vi "对中台复检判定.vi"(7 "Result":refnum<vi>, 10 "判定参数":T1={"主副信号和MAX"={"单位"="", "下限"=0.0, "上限"=0.0}, "主副信号和MIN"={"单位"="", "下限"=0.0, "上限"=0.0}, "主信号线性误差"={"单位"="", "下限"=0.0, "上限"=0.0}, "副信号线性误差"={"单位"="", "下限"=0.0, "上限"=0.0}, "主信号MAX"={"单位"="", "下限"=0.0, "上限"=0.0}, "主信号MIN"={"单位"="", "下限"=0.0, "上限"=0.0}, "副信号MAX"={"单位"="", "下限"=0.0, "上限"=0.0}, "副信号MIN"={"单位"="", "下限"=0.0, "上限"=0.0}, "中心偏移量"={"单位"="", "下限"=0.0, "上限"=0.0}, "定点设置"={"单位"="", "下限"=20.0, "上限"=30.0}, "定点左侧主信号"={"单位"="", "下限"=0.0, "上限"=0.0}, "定点左侧副信号"={"单位"="", "下限"=0.0, "上限"=0.0}, "定点右侧主信号"={"单位"="", "下限"=0.0, "上限"=0.0}, "定点右侧副信号"={"单位"="", "下限"=0.0, "上限"=0.0}, "监测点1主信号滞后"={"单位"="", "下限"=0.0, "上限"=0.0}, "监测点1副信号滞后"={"单位"="", "下限"=0.0, "上限"=0.0}, "监测点2主信号滞后"={"单位"="", "下限"=0.0, "上限"=0.0}, "监测点2副信号滞后"={"单位"="", "下限"=0.0, "上限"=0.0}, "监测点3主信号滞后"={"单位"="", "下限"=0.0, "上限"=0.0}, "监测点3副信号滞后"={"单位"="", "下限"=0.0, "上限"=0.0}}, 11 "XY曲线":cluster{"X":dbl[], "Y":dbl[]}[](array[cluster])) -> (3 "OK？":bool)   [LabVIEW 2020]
uses:
  <vilib>/Analysis/6fits.llb/Curve Fitting Criteria.ctl
  Global_Variable/Global.vi
  <vilib>/Analysis/NI_AALPro.lvlib
  <vilib>/Analysis/NI_AAL_Geometry.lvlib
panel:
  out "定点设置":dbl
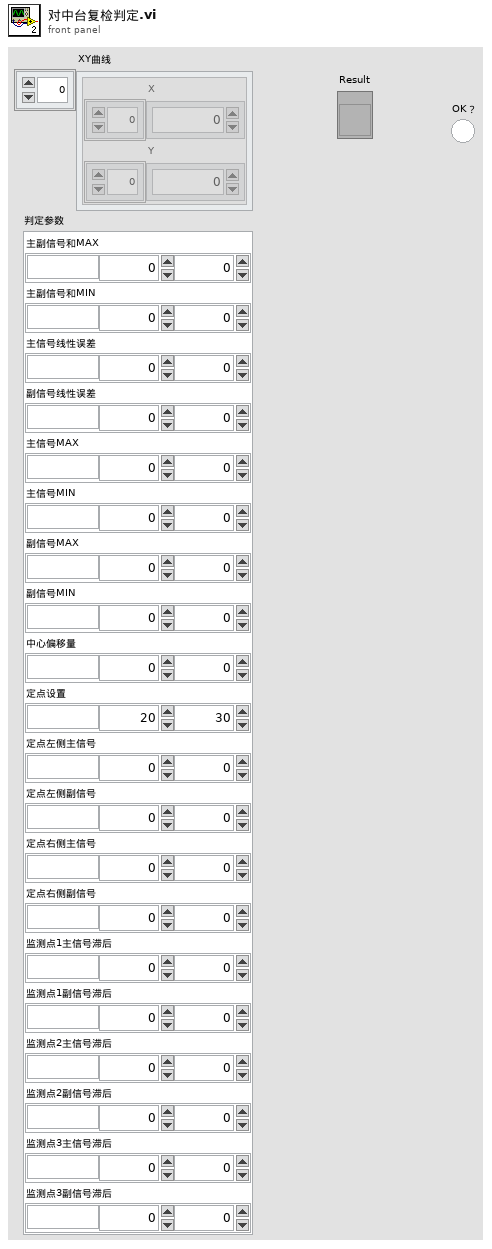
[diagram p1: front panel]
types:
  T1 = cluster{"主副信号和MAX":cluster{"单位":string, "下限":dbl, "上限":dbl}, "主副信号和MIN":cluster{"单位":string, "下限":dbl, "上限":dbl}, "主信号线性误差":cluster{"单位":string, "下限":dbl, "上限":dbl}, "副信号线性误差":cluster{"单位":string, "下限":dbl, "上限":dbl}, "主信号MAX":cluster{"单位":string, "下限":dbl, "上限":dbl}, "主信号MIN":cluster{"单位":string, "下限":dbl, "上限":dbl}, "副信号MAX":cluster{"单位":string, "下限":dbl, "上限":dbl}, "副信号MIN":cluster{"单位":string, "下限":dbl, "上限":dbl}, "中心偏移量":cluster{"单位":string, "下限":dbl, "上限":dbl}, "定点设置":cluster{"单位":string, "下限":dbl, "上限":dbl}, "定点左侧主信号":cluster{"单位":string, "下限":dbl, "上限":dbl}, "定点左侧副信号":cluster{"单位":string, "下限":dbl, "上限":dbl}, "定点右侧主信号":cluster{"单位":string, "下限":dbl, "上限":dbl}, "定点右侧副信号":cluster{"单位":string, "下限":dbl, "上限":dbl}, "监测点1主信号滞后":cluster{"单位":string, "下限":dbl, "上限":dbl}, "监测点1副信号滞后":cluster{"单位":string, "下限":dbl, "上限":dbl}, "监测点2主信号滞后":cluster{"单位":string, "下限":dbl, "上限":dbl}, "监测点2副信号滞后":cluster{"单位":string, "下限":dbl, "上限":dbl}, "监测点3主信号滞后":cluster{"单位":string, "下限":dbl, "上限":dbl}, "监测点3副信号滞后":cluster{"单位":string, "下限":dbl, "上限":dbl}}
  T2 = typedef "NI_AALPro.lvlib/Curve Fitting Criteria.ctl" = u16
  T3 = cluster{"复检速度":dbl, "换向扭矩":dbl, "判定范围下限":dbl, "判定范围上限":dbl, "滞后监测点1":dbl, "滞后监测点2":dbl, "滞后监测点3":dbl}
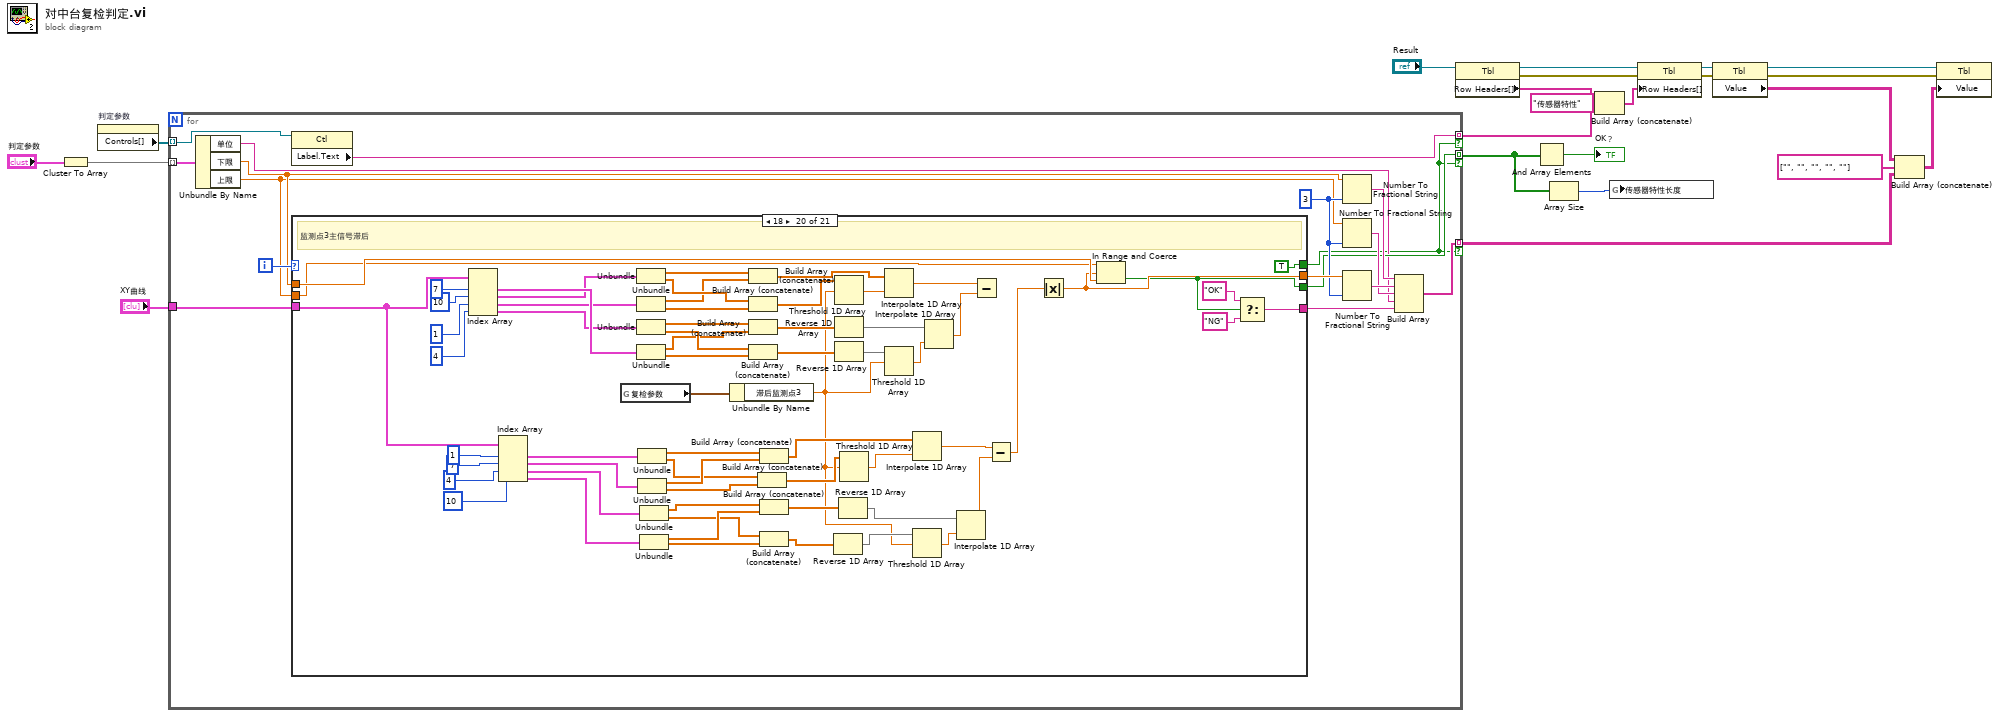
[diagram p0: block diagram]
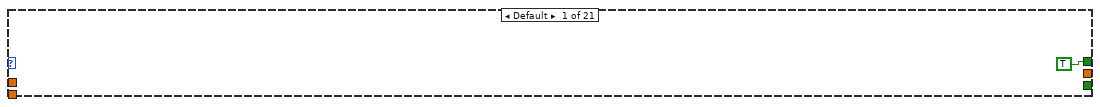
[diagram p2: hidden frame]
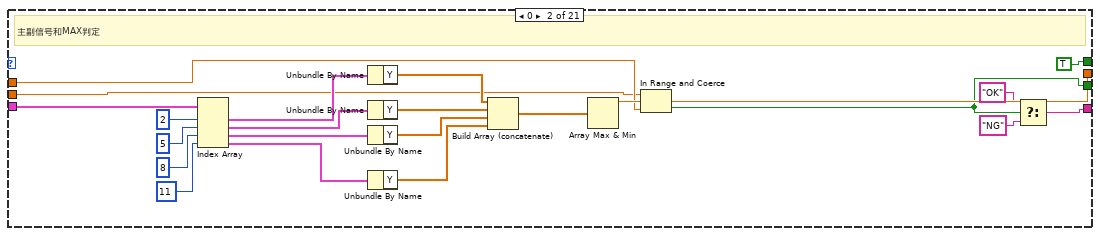
[diagram p3: hidden frame]
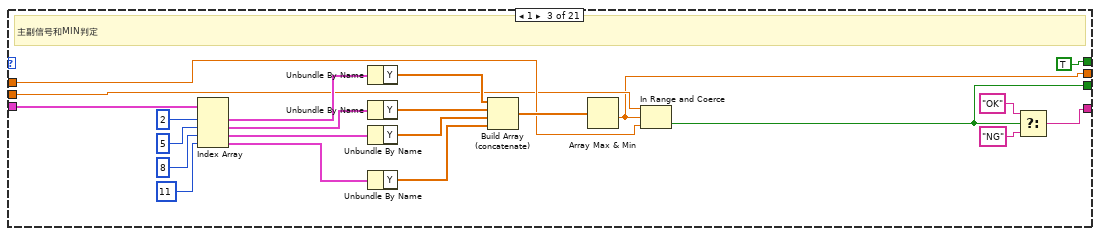
[diagram p4: hidden frame]
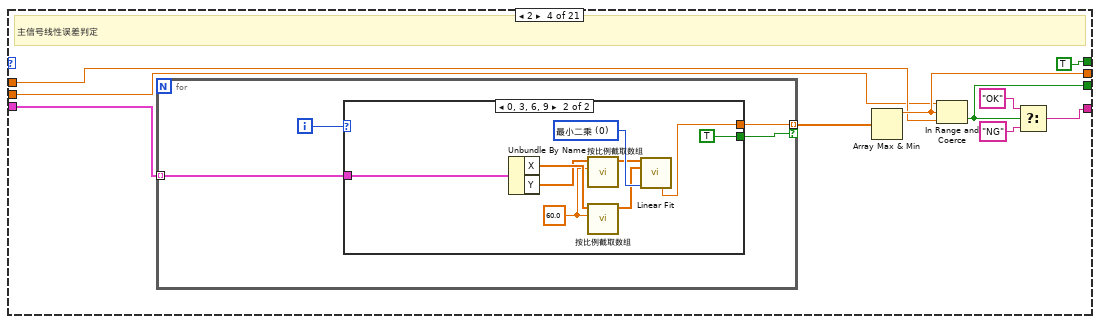
[diagram p5: hidden frame]
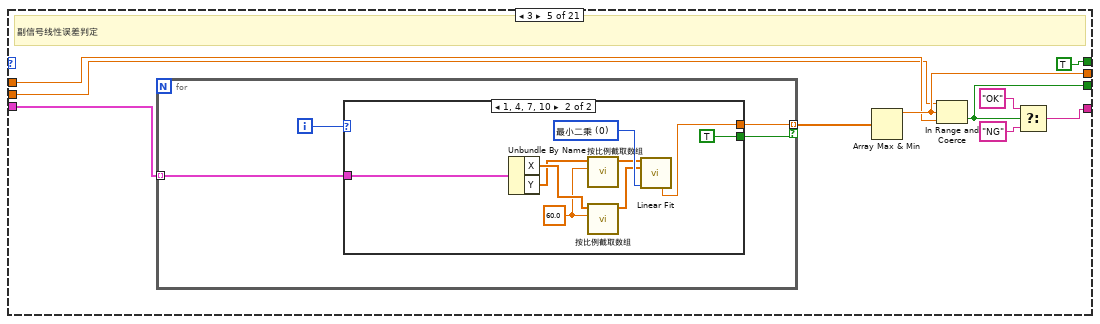
[diagram p7: hidden frame]
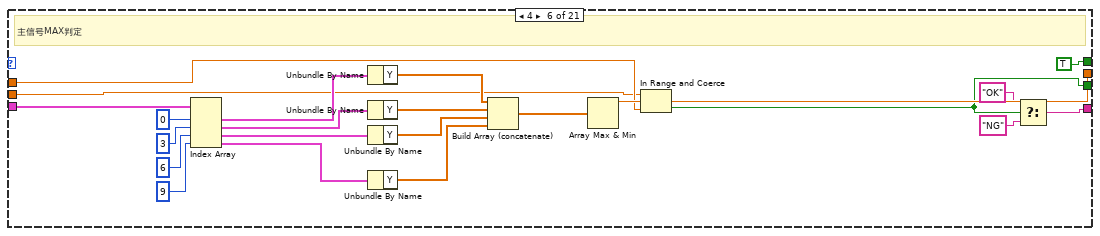
[diagram p9: hidden frame]
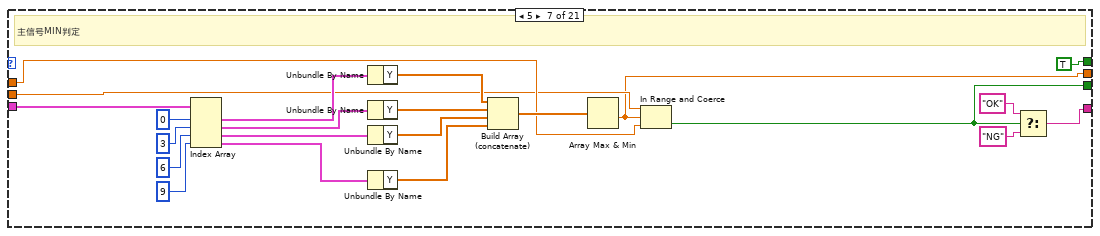
[diagram p10: hidden frame]
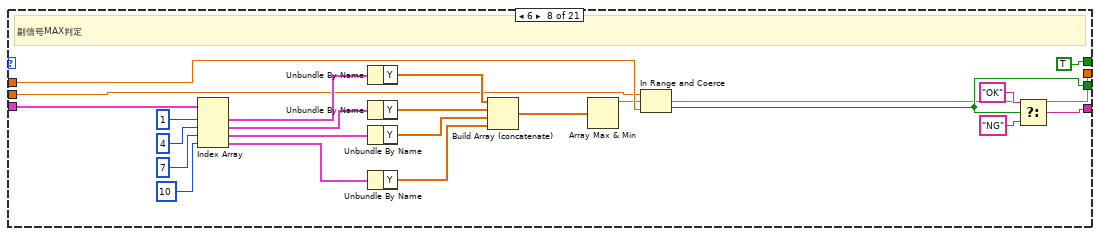
[diagram p11: hidden frame]
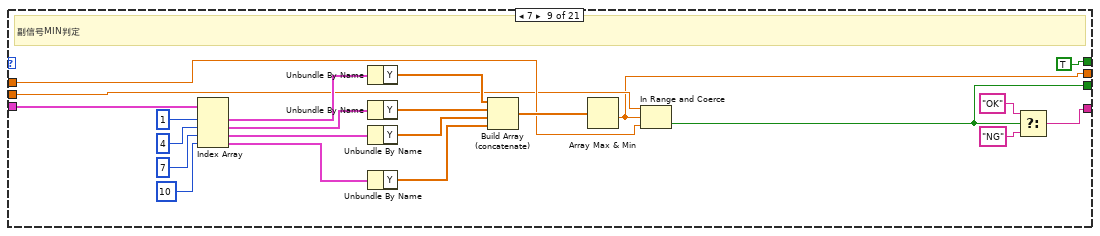
[diagram p12: hidden frame]
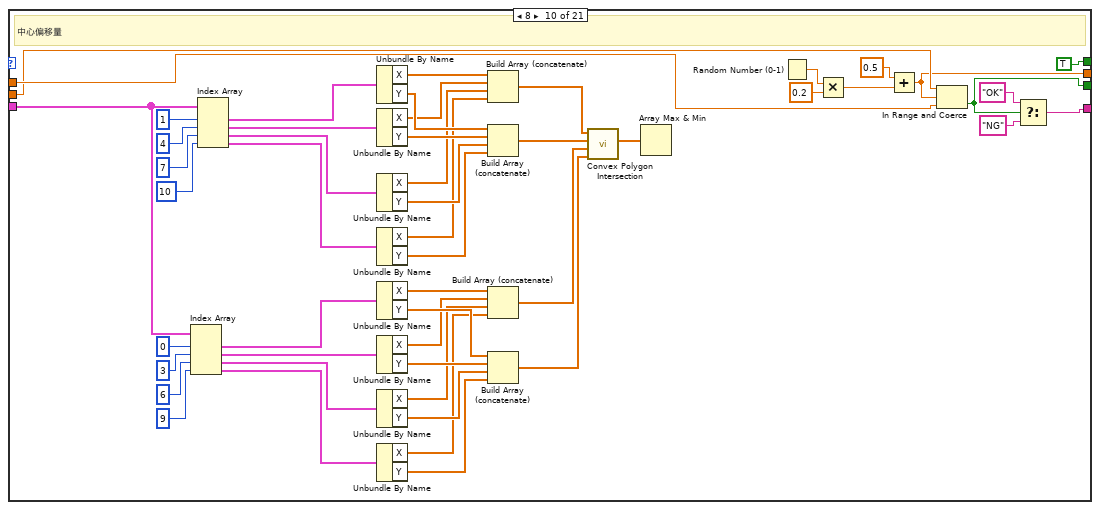
[diagram p13: hidden frame]
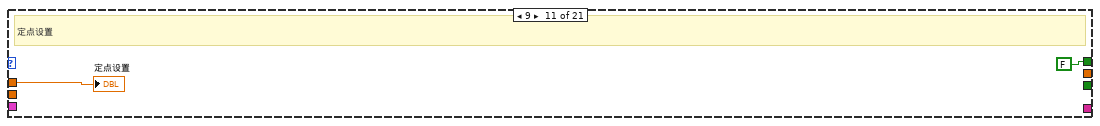
[diagram p14: hidden frame]
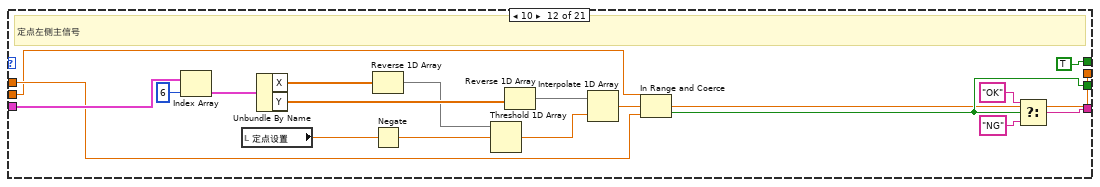
[diagram p15: hidden frame]
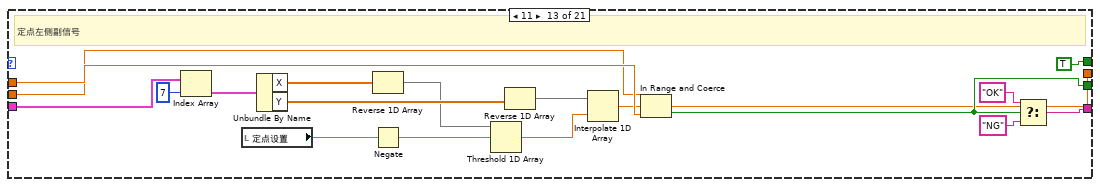
[diagram p16: hidden frame]
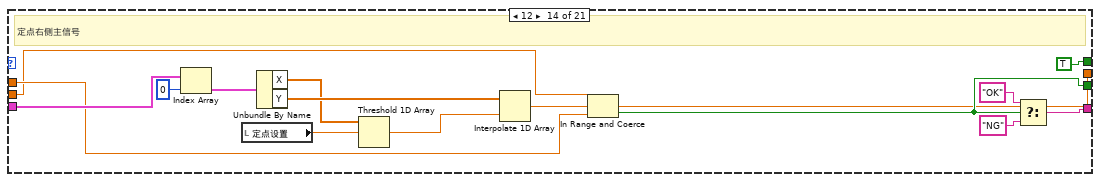
[diagram p17: hidden frame]
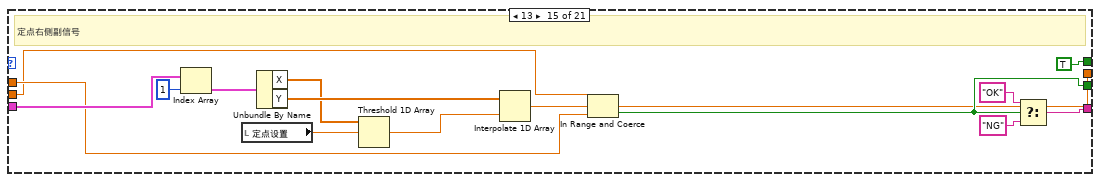
[diagram p18: hidden frame]
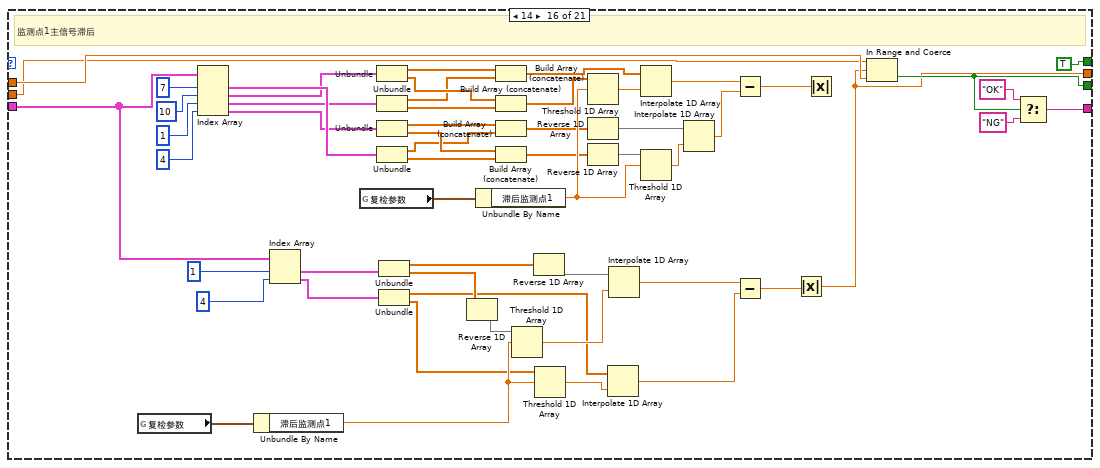
[diagram p19: hidden frame]
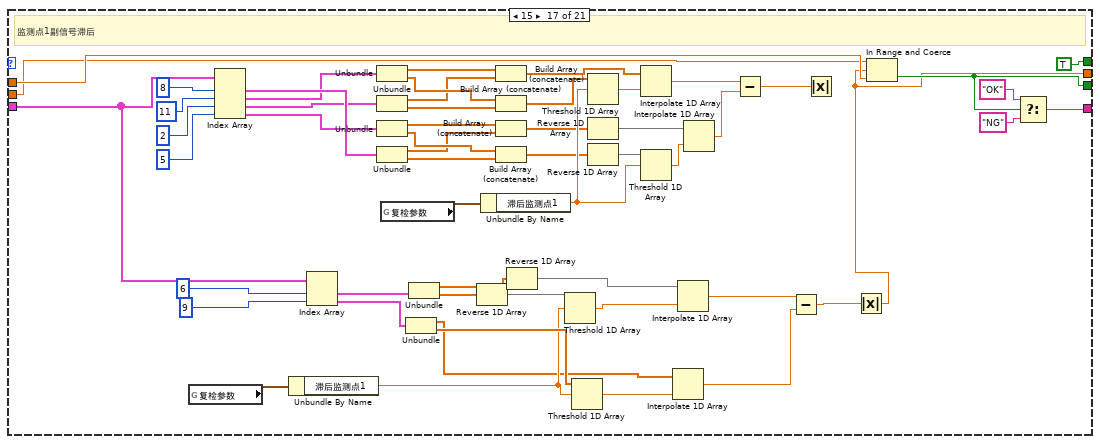
[diagram p20: hidden frame]
diagram:
  n1 = Cluster To Array(cluster="判定参数") -> (array=w22:cluster{"单位":string, "下限":dbl, "上限":dbl}[])
  n2 = property on="判定参数" class="Clust (严格)"() -> ("Controls[]"=w20:refnum<vi>[])  [unwired: 2 in, 2 out]
  n3 = for {
    tunnel: w22 -> [w39] mode=indexing
    tunnel: w20 -> [w37] mode=indexing
    tunnel: "XY曲线" -> [w35]
    tunnel: [w29] -> w2 mode=indexing if=w23
    tunnel: [w25] -> w4 mode=indexing if=w23
    tunnel: [w24] -> w8 mode=indexing if=w23
    i -> [w38]
    w34 = i16 3 ("精度(6)")
    n4 = Unbundle By Name(w39) -> ("单位"=w28:string, "下限"=w27:dbl, "上限"=w26:dbl)
    n5 = property class="Ctl"(reference=w37) -> ("Label.Text"=w24:string)  [unwired: 1 in, 2 out]
    n6 = case shown="18" w38 {
      tunnel: [_ w48 w63 w94 w117 w138 w154 w176 w198 w219 _ w275 w292 w309 w324 w340 w392 w447 w500 w607 w643] -> w36
      tunnel: w35 -> [_ w62 w84 w86 w109 w152 w174 w196 w218 w237 _ w288 w306 w321 w336 w355 w410 w457 w504 w581 w621]
      tunnel: [_ w45 w68 w91 w114 w135 w158 w180 w202 w254 _ w284 w302 w317 w332 w377 w432 w486 w539 w603 w639] -> w30
      tunnel: [_ w44 w67 w90 w113 w134 w157 w179 w201 w253 _ w283 w301 w316 w331 w378 w433 w487 w540 w604 w640] -> w29
      tunnel: w27 -> [_ w43 w66 w89 w112 w133 w156 w178 w200 w252 w269 w282 w300 w315 w330 w382 w437 w491 w544 w609 w645]
      tunnel: w26 -> [_ w42 w65 w88 w111 w132 w155 w177 w199 w251 _ w281 w299 w314 w329 w381 w436 w490 w543 w608 w644]
      tunnel: [TRUE TRUE TRUE TRUE TRUE TRUE TRUE TRUE TRUE TRUE FALSE TRUE TRUE TRUE TRUE TRUE TRUE TRUE TRUE TRUE TRUE] -> w23
      frame Default {
      }
      frame 0 {
        # "主副信号和MAX判定"
        n7 = Index Array(array=w62, index #1=2 ("索引"), index #2=5 ("索引"), index #3=8 ("索引"), index #4=11 ("索引")) -> (element #1=w57:cluster{"X":dbl[], "Y":dbl[]}, element #2=w54:cluster{"X":dbl[], "Y":dbl[]}, element #3=w55:cluster{"X":dbl[], "Y":dbl[]}, element #4=w56:cluster{"X":dbl[], "Y":dbl[]})
        n8 = Unbundle By Name(w57) -> ("Y"=w53:dbl[])
        n9 = Unbundle By Name(w54) -> ("Y"=w52:dbl[])
        n10 = Unbundle By Name(w55) -> ("Y"=w51:dbl[])
        n11 = Unbundle By Name(w56) -> ("Y"=w50:dbl[])
        n12 = Build Array (concatenate)(w53, w52, w51, w50) -> (w49:dbl[])
        n13 = Array Max & Min(array=w49) -> (max value=w48:dbl)  [unwired: 3 out]
        n14 = In Range and Coerce(upper limit=w42, x=w48, lower limit=w43) -> (In Range?=w44:bool)  [unwired: 1 out]
        n15 = Select(t="OK", s=w44, f="NG") -> (s? t:f=w45:string)
      }
      frame 1 {
        # "主副信号和MIN判定"
        n16 = Index Array(array=w84, index #1=2 ("索引"), index #2=5 ("索引"), index #3=8 ("索引"), index #4=11 ("索引")) -> (element #1=w79:cluster{"X":dbl[], "Y":dbl[]}, element #2=w76:cluster{"X":dbl[], "Y":dbl[]}, element #3=w77:cluster{"X":dbl[], "Y":dbl[]}, element #4=w78:cluster{"X":dbl[], "Y":dbl[]})
        n17 = Unbundle By Name(w79) -> ("Y"=w75:dbl[])
        n18 = Unbundle By Name(w76) -> ("Y"=w74:dbl[])
        n19 = Unbundle By Name(w77) -> ("Y"=w73:dbl[])
        n20 = Unbundle By Name(w78) -> ("Y"=w72:dbl[])
        n21 = Build Array (concatenate)(w75, w74, w73, w72) -> (w71:dbl[])
        n22 = Array Max & Min(array=w71) -> (min value=w63:dbl)  [unwired: 3 out]
        n23 = In Range and Coerce(upper limit=w65, x=w63, lower limit=w66) -> (In Range?=w67:bool)  [unwired: 1 out]
        n24 = Select(t="OK", s=w67, f="NG") -> (s? t:f=w68:string)
      }
      frame 2 {
        # "主信号线性误差判定"
        n25 = for {
          tunnel: w86 -> [w97] mode=indexing
          tunnel: [w96] -> w85 mode=indexing if=w95
          i -> [w98]
          n26 = case shown="0, 3, 6, 9" w98 {
            tunnel: w97 -> [_ w107]
            tunnel: [_ w105] -> w96
            tunnel: [_ TRUE] -> w95
            frame Default {
            }
            frame 0, 3, 6, 9 {
              w99 = 60.0 ("长度")
              w106 = T2 0 items=["最小二乘", "最小绝对残差", "Bisquare"] ("method")
              n27 = Unbundle By Name(w107) -> ("X"=w103:dbl[], "Y"=w101:dbl[])
              n28 = call "按比例截取数组.vi"("长度"=w99, "X"=w101) -> ("Y"=w100:dbl[])  [unwired: 9 in]
              n29 = call "按比例截取数组.vi"("长度"=w99, "X"=w103) -> ("Y"=w102:dbl[])  [unwired: 9 in]
              n30 = call <vilib>:"Linear Fit.vi"("Y"=w100, "X"=w102, "method"=w106) -> ("residue"=w105:dbl)  [unwired: 8 in, 4 out]
            }
          }
        }
        n31 = Array Max & Min(array=w85) -> (max value=w94:dbl)  [unwired: 3 out]
        n32 = In Range and Coerce(upper limit=w88, x=w94, lower limit=w89) -> (In Range?=w90:bool)  [unwired: 1 out]
        n33 = Select(t="OK", s=w90, f="NG") -> (s? t:f=w91:string)
      }
      frame 3 {
        # "副信号线性误差判定"
        n34 = for {
          tunnel: w109 -> [w120] mode=indexing
          tunnel: [w119] -> w108 mode=indexing if=w118
          i -> [w121]
          n35 = case shown="1, 4, 7, 10" w121 {
            tunnel: w120 -> [_ w130]
            tunnel: [_ w128] -> w119
            tunnel: [_ TRUE] -> w118
            frame Default {
            }
            frame 1, 4, 7, 10 {
              w122 = 60.0 ("长度")
              w129 = T2 0 items=["最小二乘", "最小绝对残差", "Bisquare"] ("method")
              n36 = Unbundle By Name(w130) -> ("X"=w126:dbl[], "Y"=w124:dbl[])
              n37 = call "按比例截取数组.vi"("长度"=w122, "X"=w124) -> ("Y"=w123:dbl[])  [unwired: 9 in]
              n38 = call "按比例截取数组.vi"("长度"=w122, "X"=w126) -> ("Y"=w125:dbl[])  [unwired: 9 in]
              n39 = call <vilib>:"Linear Fit.vi"("Y"=w123, "X"=w125, "method"=w129) -> ("residue"=w128:dbl)  [unwired: 8 in, 4 out]
            }
          }
        }
        n40 = Array Max & Min(array=w108) -> (max value=w117:dbl)  [unwired: 3 out]
        n41 = In Range and Coerce(upper limit=w111, x=w117, lower limit=w112) -> (In Range?=w113:bool)  [unwired: 1 out]
        n42 = Select(t="OK", s=w113, f="NG") -> (s? t:f=w114:string)
      }
      frame 4 {
        # "主信号MAX判定"
        n43 = Index Array(array=w152, index #1=0 ("索引"), index #2=3 ("索引"), index #3=6 ("索引"), index #4=9 ("索引")) -> (element #1=w147:cluster{"X":dbl[], "Y":dbl[]}, element #2=w144:cluster{"X":dbl[], "Y":dbl[]}, element #3=w145:cluster{"X":dbl[], "Y":dbl[]}, element #4=w146:cluster{"X":dbl[], "Y":dbl[]})
        n44 = Unbundle By Name(w147) -> ("Y"=w143:dbl[])
        n45 = Unbundle By Name(w144) -> ("Y"=w142:dbl[])
        n46 = Unbundle By Name(w145) -> ("Y"=w141:dbl[])
        n47 = Unbundle By Name(w146) -> ("Y"=w140:dbl[])
        n48 = Build Array (concatenate)(w143, w142, w141, w140) -> (w139:dbl[])
        n49 = Array Max & Min(array=w139) -> (max value=w138:dbl)  [unwired: 3 out]
        n50 = In Range and Coerce(upper limit=w132, x=w138, lower limit=w133) -> (In Range?=w134:bool)  [unwired: 1 out]
        n51 = Select(t="OK", s=w134, f="NG") -> (s? t:f=w135:string)
      }
      frame 5 {
        # "主信号MIN判定"
        n52 = Index Array(array=w174, index #1=0 ("索引"), index #2=3 ("索引"), index #3=6 ("索引"), index #4=9 ("索引")) -> (element #1=w169:cluster{"X":dbl[], "Y":dbl[]}, element #2=w166:cluster{"X":dbl[], "Y":dbl[]}, element #3=w167:cluster{"X":dbl[], "Y":dbl[]}, element #4=w168:cluster{"X":dbl[], "Y":dbl[]})
        n53 = Unbundle By Name(w169) -> ("Y"=w165:dbl[])
        n54 = Unbundle By Name(w166) -> ("Y"=w164:dbl[])
        n55 = Unbundle By Name(w167) -> ("Y"=w163:dbl[])
        n56 = Unbundle By Name(w168) -> ("Y"=w162:dbl[])
        n57 = Build Array (concatenate)(w165, w164, w163, w162) -> (w161:dbl[])
        n58 = Array Max & Min(array=w161) -> (min value=w154:dbl)  [unwired: 3 out]
        n59 = In Range and Coerce(upper limit=w155, x=w154, lower limit=w156) -> (In Range?=w157:bool)  [unwired: 1 out]
        n60 = Select(t="OK", s=w157, f="NG") -> (s? t:f=w158:string)
      }
      frame 6 {
        # "副信号MAX判定"
        n61 = Index Array(array=w196, index #1=1 ("索引"), index #2=4 ("索引"), index #3=7 ("索引"), index #4=10 ("索引")) -> (element #1=w191:cluster{"X":dbl[], "Y":dbl[]}, element #2=w188:cluster{"X":dbl[], "Y":dbl[]}, element #3=w189:cluster{"X":dbl[], "Y":dbl[]}, element #4=w190:cluster{"X":dbl[], "Y":dbl[]})
        n62 = Unbundle By Name(w191) -> ("Y"=w187:dbl[])
        n63 = Unbundle By Name(w188) -> ("Y"=w186:dbl[])
        n64 = Unbundle By Name(w189) -> ("Y"=w185:dbl[])
        n65 = Unbundle By Name(w190) -> ("Y"=w184:dbl[])
        n66 = Build Array (concatenate)(w187, w186, w185, w184) -> (w183:dbl[])
        n67 = Array Max & Min(array=w183) -> (max value=w176:dbl)  [unwired: 3 out]
        n68 = In Range and Coerce(upper limit=w177, x=w176, lower limit=w178) -> (In Range?=w179:bool)  [unwired: 1 out]
        n69 = Select(t="OK", s=w179, f="NG") -> (s? t:f=w180:string)
      }
      frame 7 {
        # "副信号MIN判定"
        n70 = Index Array(array=w218, index #1=1 ("索引"), index #2=4 ("索引"), index #3=7 ("索引"), index #4=10 ("索引")) -> (element #1=w213:cluster{"X":dbl[], "Y":dbl[]}, element #2=w210:cluster{"X":dbl[], "Y":dbl[]}, element #3=w211:cluster{"X":dbl[], "Y":dbl[]}, element #4=w212:cluster{"X":dbl[], "Y":dbl[]})
        n71 = Unbundle By Name(w213) -> ("Y"=w209:dbl[])
        n72 = Unbundle By Name(w210) -> ("Y"=w208:dbl[])
        n73 = Unbundle By Name(w211) -> ("Y"=w207:dbl[])
        n74 = Unbundle By Name(w212) -> ("Y"=w206:dbl[])
        n75 = Build Array (concatenate)(w209, w208, w207, w206) -> (w205:dbl[])
        n76 = Array Max & Min(array=w205) -> (min value=w198:dbl)  [unwired: 3 out]
        n77 = In Range and Coerce(upper limit=w199, x=w198, lower limit=w200) -> (In Range?=w201:bool)  [unwired: 1 out]
        n78 = Select(t="OK", s=w201, f="NG") -> (s? t:f=w202:string)
      }
      frame 8 {
        # "中心偏移量"
        n79 = Index Array(array=w237, index #1=0 ("索引"), index #2=3 ("索引"), index #3=6 ("索引"), index #4=9 ("索引")) -> (element #1=w264:cluster{"X":dbl[], "Y":dbl[]}, element #2=w261:cluster{"X":dbl[], "Y":dbl[]}, element #3=w262:cluster{"X":dbl[], "Y":dbl[]}, element #4=w263:cluster{"X":dbl[], "Y":dbl[]})
        n80 = Index Array(array=w237, index #1=1 ("索引"), index #2=4 ("索引"), index #3=7 ("索引"), index #4=10 ("索引")) -> (element #1=w242:cluster{"X":dbl[], "Y":dbl[]}, element #2=w245:cluster{"X":dbl[], "Y":dbl[]}, element #3=w244:cluster{"X":dbl[], "Y":dbl[]}, element #4=w243:cluster{"X":dbl[], "Y":dbl[]})
        n81 = Unbundle By Name(w242) -> ("X"=w236:dbl[], "Y"=w246:dbl[])
        n82 = Unbundle By Name(w245) -> ("X"=w235:dbl[], "Y"=w247:dbl[])
        n83 = Unbundle By Name(w244) -> ("X"=w234:dbl[], "Y"=w248:dbl[])
        n84 = Unbundle By Name(w243) -> ("X"=w233:dbl[], "Y"=w249:dbl[])
        n85 = Unbundle By Name(w264) -> ("X"=w232:dbl[], "Y"=w260:dbl[])
        n86 = Unbundle By Name(w261) -> ("X"=w231:dbl[], "Y"=w259:dbl[])
        n87 = Unbundle By Name(w262) -> ("X"=w230:dbl[], "Y"=w258:dbl[])
        n88 = Unbundle By Name(w263) -> ("X"=w229:dbl[], "Y"=w257:dbl[])
        n89 = Build Array (concatenate)(w236, w235, w234, w233) -> (w226:dbl[])
        n90 = Build Array (concatenate)(w246, w247, w248, w249) -> (w228:dbl[])
        n91 = Build Array (concatenate)(w232, w231, w230, w229) -> (w225:dbl[])
        n92 = Build Array (concatenate)(w260, w259, w258, w257) -> (w224:dbl[])
        n93 = call <vilib>:"Convex Polygon Intersection.vi"("Y 2"=w224, "X 2"=w225, "Y 1"=w228, "X 1"=w226) -> ("Intersection Y"=w227:dbl[])  [unwired: 5 in, 2 out]
        n94 = Array Max & Min(array=w227) -> ()  [unwired: 4 out]
        n95 = Random Number (0-1)() -> (number: 0 to 1=w222:dbl)
        n96 = Multiply(x=w222, y=0.2) -> (x*y=w220:dbl)
        n97 = Add(x=0.5, y=w220) -> (x+y=w219:dbl)
        n98 = In Range and Coerce(upper limit=w251, x=w219, lower limit=w252) -> (In Range?=w253:bool)  [unwired: 1 out]
        n99 = Select(t="OK", s=w253, f="NG") -> (s? t:f=w254:string)
      }
      frame 9 {
        # "定点设置"
        "定点设置" <- w269
      }
      frame 10 {
        # "定点左侧主信号"
        n100 = Index Array(array=w288, index=6 ("索引")) -> (element=w287:cluster{"X":dbl[], "Y":dbl[]})
        n101 = local read "定点设置"() -> (w277:dbl)
        n102 = Unbundle By Name(w287) -> ("X"=w274:dbl[], "Y"=w276:dbl[])
        n103 = Reverse 1D Array(array=w274) -> (reversed array=w272:dbl[])
        n104 = Negate(x=w277) -> (-x=w273:dbl)
        n105 = Threshold 1D Array(2:w273, 3:w272) -> (0:w278:dbl)  [unwired: 1 in]
        n106 = Reverse 1D Array(array=w276) -> (reversed array=w271:dbl[])
        n107 = Interpolate 1D Array(1:w278, 2:w271) -> (0:w275:dbl)
        n108 = In Range and Coerce(upper limit=w281, x=w275, lower limit=w282) -> (In Range?=w283:bool)  [unwired: 1 out]
        n109 = Select(t="OK", s=w283, f="NG") -> (s? t:f=w284:string)
      }
      frame 11 {
        # "定点左侧副信号"
        n110 = Index Array(array=w306, index=7 ("索引")) -> (element=w305:cluster{"X":dbl[], "Y":dbl[]})
        n111 = local read "定点设置"() -> (w294:dbl)
        n112 = Unbundle By Name(w305) -> ("X"=w295:dbl[], "Y"=w293:dbl[])
        n113 = Reverse 1D Array(array=w295) -> (reversed array=w291:dbl[])
        n114 = Negate(x=w294) -> (-x=w289:dbl)
        n115 = Threshold 1D Array(2:w289, 3:w291) -> (0:w296:dbl)  [unwired: 1 in]
        n116 = Reverse 1D Array(array=w293) -> (reversed array=w290:dbl[])
        n117 = Interpolate 1D Array(1:w296, 2:w290) -> (0:w292:dbl)
        n118 = In Range and Coerce(upper limit=w299, x=w292, lower limit=w300) -> (In Range?=w301:bool)  [unwired: 1 out]
        n119 = Select(t="OK", s=w301, f="NG") -> (s? t:f=w302:string)
      }
      frame 12 {
        # "定点右侧主信号"
        n120 = Index Array(array=w321, index=0 ("索引")) -> (element=w320:cluster{"X":dbl[], "Y":dbl[]})
        n121 = local read "定点设置"() -> (w307:dbl)
        n122 = Unbundle By Name(w320) -> ("X"=w308:dbl[], "Y"=w310:dbl[])
        n123 = Threshold 1D Array(2:w307, 3:w308) -> (0:w311:dbl)  [unwired: 1 in]
        n124 = Interpolate 1D Array(1:w311, 2:w310) -> (0:w309:dbl)
        n125 = In Range and Coerce(upper limit=w314, x=w309, lower limit=w315) -> (In Range?=w316:bool)  [unwired: 1 out]
        n126 = Select(t="OK", s=w316, f="NG") -> (s? t:f=w317:string)
      }
      frame 13 {
        # "定点右侧副信号"
        n127 = Index Array(array=w336, index=1 ("索引")) -> (element=w335:cluster{"X":dbl[], "Y":dbl[]})
        n128 = local read "定点设置"() -> (w322:dbl)
        n129 = Unbundle By Name(w335) -> ("X"=w323:dbl[], "Y"=w325:dbl[])
        n130 = Threshold 1D Array(2:w322, 3:w323) -> (0:w326:dbl)  [unwired: 1 in]
        n131 = Interpolate 1D Array(1:w326, 2:w325) -> (0:w324:dbl)
        n132 = In Range and Coerce(upper limit=w329, x=w324, lower limit=w330) -> (In Range?=w331:bool)  [unwired: 1 out]
        n133 = Select(t="OK", s=w331, f="NG") -> (s? t:f=w332:string)
      }
      frame 14 {
        # "监测点1主信号滞后"
        n134 = global read "Global.vi" "复检参数"() -> (w350:T3)
        n135 = Index Array(array=w355, index #1=7 ("索引"), index #2=10 ("索引"), index #3=1 ("索引"), index #4=4 ("索引")) -> (element #1=w373:cluster{"X":dbl[], "Y":dbl[]}, element #2=w372:cluster{"X":dbl[], "Y":dbl[]}, element #3=w369:cluster{"X":dbl[], "Y":dbl[]}, element #4=w368:cluster{"X":dbl[], "Y":dbl[]})
        n136 = Unbundle By Name(w350) -> ("滞后监测点1"=w347:dbl)
        n137 = Index Array(array=w355, index #1=1 ("索引"), index #2=4 ("索引")) -> (element #1=w352:cluster{"X":dbl[], "Y":dbl[]}, element #2=w351:cluster{"X":dbl[], "Y":dbl[]})
        n138 = global read "Global.vi" "复检参数"() -> (w391:T3)
        n139 = Unbundle(w372) -> ("X"=w367:dbl[], "Y"=w366:dbl[])
        n140 = Unbundle(w369) -> ("X"=w365:dbl[], "Y"=w364:dbl[])
        n141 = Unbundle(w368) -> ("X"=w363:dbl[], "Y"=w362:dbl[])
        n142 = Unbundle(w373) -> ("X"=w361:dbl[], "Y"=w360:dbl[])
        n143 = Unbundle(w352) -> ("X"=w343:dbl[], "Y"=w342:dbl[])
        n144 = Unbundle(w351) -> ("X"=w339:dbl[], "Y"=w341:dbl[])
        n145 = Reverse 1D Array(array=w342) -> (reversed array=w337:dbl[])
        n146 = Unbundle By Name(w391) -> ("滞后监测点1"=w388:dbl)
        n147 = Build Array (concatenate)(w367, w365) -> (w359:dbl[])
        n148 = Build Array (concatenate)(w366, w364) -> (w358:dbl[])
        n149 = Build Array (concatenate)(w363, w361) -> (w357:dbl[])
        n150 = Build Array (concatenate)(w362, w360) -> (w356:dbl[])
        n151 = Threshold 1D Array(2:w347, 3:w337) -> (0:w349:dbl)  [unwired: 1 in]
        n152 = Reverse 1D Array(array=w343) -> (reversed array=w338:dbl[])
        n153 = Threshold 1D Array(2:w347, 3:w341) -> (0:w345:dbl)  [unwired: 1 in]
        n154 = Threshold 1D Array(2:w388, 3:w358) -> (0:w390:dbl)  [unwired: 1 in]
        n155 = Reverse 1D Array(array=w357) -> (reversed array=w376:dbl[])
        n156 = Reverse 1D Array(array=w356) -> (reversed array=w389:dbl[])
        n157 = Interpolate 1D Array(1:w345, 2:w339) -> (0:w344:dbl)
        n158 = Interpolate 1D Array(1:w349, 2:w338) -> (0:w348:dbl)
        n159 = Interpolate 1D Array(1:w390, 2:w359) -> (0:w386:dbl)
        n160 = Threshold 1D Array(2:w388, 3:w389) -> (0:w387:dbl)  [unwired: 1 in]
        n161 = Interpolate 1D Array(1:w387, 2:w376) -> (0:w385:dbl)
        n162 = Subtract(x=w386, y=w385) -> (x-y=w384:dbl)
        n163 = Subtract(x=w348, y=w344) -> (x-y=w346:dbl)
        n164 = Absolute Value(x=w346) -> (abs(x)=w340:dbl)
        n165 = Absolute Value(x=w384) -> ()  [unwired: 1 out]
        n166 = In Range and Coerce(upper limit=w381, x=w340, lower limit=w382) -> (In Range?=w378:bool)  [unwired: 1 out]
        n167 = Select(t="OK", s=w378, f="NG") -> (s? t:f=w377:string)
      }
      frame 15 {
        # "监测点1副信号滞后"
        n168 = global read "Global.vi" "复检参数"() -> (w405:T3)
        n169 = Index Array(array=w410, index #1=8 ("索引"), index #2=11 ("索引"), index #3=2 ("索引"), index #4=5 ("索引")) -> (element #1=w428:cluster{"X":dbl[], "Y":dbl[]}, element #2=w427:cluster{"X":dbl[], "Y":dbl[]}, element #3=w424:cluster{"X":dbl[], "Y":dbl[]}, element #4=w423:cluster{"X":dbl[], "Y":dbl[]})
        n170 = Unbundle By Name(w405) -> ("滞后监测点1"=w399:dbl)
        n171 = Index Array(array=w410, index #1=6 ("索引"), index #2=9 ("索引")) -> (element #1=w407:cluster{"X":dbl[], "Y":dbl[]}, element #2=w406:cluster{"X":dbl[], "Y":dbl[]})
        n172 = Unbundle(w427) -> ("X"=w422:dbl[], "Y"=w421:dbl[])
        n173 = Unbundle(w424) -> ("X"=w420:dbl[], "Y"=w419:dbl[])
        n174 = Unbundle(w423) -> ("X"=w418:dbl[], "Y"=w417:dbl[])
        n175 = Unbundle(w428) -> ("X"=w416:dbl[], "Y"=w415:dbl[])
        n176 = global read "Global.vi" "复检参数"() -> (w446:T3)
        n177 = Unbundle(w406) -> ("X"=w395:dbl[], "Y"=w400:dbl[])
        n178 = Unbundle(w407) -> ("X"=w403:dbl[], "Y"=w404:dbl[])
        n179 = Reverse 1D Array(array=w404) -> (reversed array=w393:dbl[])
        n180 = Unbundle By Name(w446) -> ("滞后监测点1"=w443:dbl)
        n181 = Build Array (concatenate)(w422, w420) -> (w414:dbl[])
        n182 = Build Array (concatenate)(w421, w419) -> (w413:dbl[])
        n183 = Build Array (concatenate)(w418, w416) -> (w412:dbl[])
        n184 = Build Array (concatenate)(w417, w415) -> (w411:dbl[])
        n185 = Reverse 1D Array(array=w403) -> (reversed array=w394:dbl[])
        n186 = Threshold 1D Array(2:w399, 3:w393) -> (0:w402:dbl)  [unwired: 1 in]
        n187 = Threshold 1D Array(2:w399, 3:w400) -> (0:w398:dbl)  [unwired: 1 in]
        n188 = Threshold 1D Array(2:w443, 3:w413) -> (0:w445:dbl)  [unwired: 1 in]
        n189 = Reverse 1D Array(array=w412) -> (reversed array=w431:dbl[])
        n190 = Reverse 1D Array(array=w411) -> (reversed array=w444:dbl[])
        n191 = Interpolate 1D Array(1:w445, 2:w414) -> (0:w441:dbl)
        n192 = Threshold 1D Array(2:w443, 3:w444) -> (0:w442:dbl)  [unwired: 1 in]
        n193 = Interpolate 1D Array(1:w398, 2:w395) -> (0:w397:dbl)
        n194 = Interpolate 1D Array(1:w402, 2:w394) -> (0:w401:dbl)
        n195 = Interpolate 1D Array(1:w442, 2:w431) -> (0:w440:dbl)
        n196 = Subtract(x=w441, y=w440) -> (x-y=w439:dbl)
        n197 = Subtract(x=w401, y=w397) -> (x-y=w396:dbl)
        n198 = Absolute Value(x=w439) -> ()  [unwired: 1 out]
        n199 = Absolute Value(x=w396) -> (abs(x)=w392:dbl)
        n200 = In Range and Coerce(upper limit=w436, x=w392, lower limit=w437) -> (In Range?=w433:bool)  [unwired: 1 out]
        n201 = Select(t="OK", s=w433, f="NG") -> (s? t:f=w432:string)
      }
      frame 16 {
        # "监测点2主信号滞后"
        n202 = Index Array(array=w457, index #1=7 ("索引"), index #2=10 ("索引"), index #3=1 ("索引"), index #4=4 ("索引")) -> (element #1=w482:cluster{"X":dbl[], "Y":dbl[]}, element #2=w481:cluster{"X":dbl[], "Y":dbl[]}, element #3=w478:cluster{"X":dbl[], "Y":dbl[]}, element #4=w477:cluster{"X":dbl[], "Y":dbl[]})
        n203 = Index Array(array=w457, index #1=7 ("索引"), index #2=10 ("索引")) -> (element #1=w456:cluster{"X":dbl[], "Y":dbl[]}, element #2=w455:cluster{"X":dbl[], "Y":dbl[]})
        n204 = global read "Global.vi" "复检参数"() -> (w499:T3)
        n205 = Unbundle(w481) -> ("X"=w476:dbl[], "Y"=w475:dbl[])
        n206 = Unbundle(w478) -> ("X"=w474:dbl[], "Y"=w473:dbl[])
        n207 = Unbundle(w477) -> ("X"=w472:dbl[], "Y"=w471:dbl[])
        n208 = Unbundle(w482) -> ("X"=w470:dbl[], "Y"=w469:dbl[])
        n209 = Unbundle(w456) -> ("X"=w450:dbl[], "Y"=w454:dbl[])
        n210 = Unbundle(w455) -> ("X"=w452:dbl[], "Y"=w453:dbl[])
        n211 = Reverse 1D Array(array=w453) -> (reversed array=w448:dbl[])
        n212 = Reverse 1D Array(array=w452) -> (reversed array=w449:dbl[])
        n213 = Unbundle By Name(w499) -> ("滞后监测点2"=w451:dbl)
        n214 = Build Array (concatenate)(w476, w474) -> (w468:dbl[])
        n215 = Build Array (concatenate)(w475, w473) -> (w467:dbl[])
        n216 = Build Array (concatenate)(w472, w470) -> (w466:dbl[])
        n217 = Build Array (concatenate)(w471, w469) -> (w465:dbl[])
        n218 = Threshold 1D Array(2:w451, 3:w454) -> (0:w462:dbl)  [unwired: 1 in]
        n219 = Threshold 1D Array(2:w451, 3:w448) -> (0:w461:dbl)  [unwired: 1 in]
        n220 = Threshold 1D Array(2:w451, 3:w467) -> (0:w498:dbl)  [unwired: 1 in]
        n221 = Reverse 1D Array(array=w466) -> (reversed array=w485:dbl[])
        n222 = Reverse 1D Array(array=w465) -> (reversed array=w497:dbl[])
        n223 = Interpolate 1D Array(1:w498, 2:w468) -> (0:w495:dbl)
        n224 = Threshold 1D Array(2:w451, 3:w497) -> (0:w496:dbl)  [unwired: 1 in]
        n225 = Interpolate 1D Array(1:w462, 2:w450) -> (0:w460:dbl)
        n226 = Interpolate 1D Array(1:w461, 2:w449) -> (0:w459:dbl)
        n227 = Interpolate 1D Array(1:w496, 2:w485) -> (0:w494:dbl)
        n228 = Subtract(x=w495, y=w494) -> (x-y=w493:dbl)
        n229 = Subtract(x=w460, y=w459) -> (x-y=w458:dbl)
        n230 = Absolute Value(x=w493) -> ()  [unwired: 1 out]
        n231 = Absolute Value(x=w458) -> (abs(x)=w447:dbl)
        n232 = In Range and Coerce(upper limit=w490, x=w447, lower limit=w491) -> (In Range?=w487:bool)  [unwired: 1 out]
        n233 = Select(t="OK", s=w487, f="NG") -> (s? t:f=w486:string)
      }
      frame 17 {
        # "监测点2副信号滞后"
        n234 = Index Array(array=w504, index #1=8 ("索引"), index #2=11 ("索引"), index #3=2 ("索引"), index #4=5 ("索引")) -> (element #1=w535:cluster{"X":dbl[], "Y":dbl[]}, element #2=w534:cluster{"X":dbl[], "Y":dbl[]}, element #3=w531:cluster{"X":dbl[], "Y":dbl[]}, element #4=w530:cluster{"X":dbl[], "Y":dbl[]})
        n235 = Index Array(array=w504, index #1=0 ("索引"), index #2=3 ("索引")) -> (element #1=w515:cluster{"X":dbl[], "Y":dbl[]}, element #2=w514:cluster{"X":dbl[], "Y":dbl[]})
        n236 = Unbundle(w515) -> ("X"=w511:dbl[], "Y"=w513:dbl[])
        n237 = Unbundle(w514) -> ("X"=w509:dbl[], "Y"=w510:dbl[])
        n238 = global read "Global.vi" "复检参数"() -> (w552:T3)
        n239 = Unbundle(w534) -> ("X"=w529:dbl[], "Y"=w528:dbl[])
        n240 = Unbundle(w531) -> ("X"=w527:dbl[], "Y"=w526:dbl[])
        n241 = Unbundle(w530) -> ("X"=w525:dbl[], "Y"=w524:dbl[])
        n242 = Unbundle(w535) -> ("X"=w523:dbl[], "Y"=w522:dbl[])
        n243 = Reverse 1D Array(array=w509) -> (reversed array=w502:dbl[])
        n244 = Reverse 1D Array(array=w510) -> (reversed array=w501:dbl[])
        n245 = Unbundle By Name(w552) -> ("滞后监测点2"=w503:dbl)
        n246 = Threshold 1D Array(2:w503, 3:w513) -> (0:w512:dbl)  [unwired: 1 in]
        n247 = Threshold 1D Array(2:w503, 3:w501) -> (0:w508:dbl)  [unwired: 1 in]
        n248 = Build Array (concatenate)(w529, w527) -> (w521:dbl[])
        n249 = Build Array (concatenate)(w528, w526) -> (w520:dbl[])
        n250 = Build Array (concatenate)(w525, w523) -> (w519:dbl[])
        n251 = Build Array (concatenate)(w524, w522) -> (w518:dbl[])
        n252 = Threshold 1D Array(2:w503, 3:w520) -> (0:w551:dbl)  [unwired: 1 in]
        n253 = Reverse 1D Array(array=w519) -> (reversed array=w538:dbl[])
        n254 = Reverse 1D Array(array=w518) -> (reversed array=w550:dbl[])
        n255 = Interpolate 1D Array(1:w512, 2:w511) -> (0:w507:dbl)
        n256 = Interpolate 1D Array(1:w508, 2:w502) -> (0:w506:dbl)
        n257 = Interpolate 1D Array(1:w551, 2:w521) -> (0:w548:dbl)
        n258 = Threshold 1D Array(2:w503, 3:w550) -> (0:w549:dbl)  [unwired: 1 in]
        n259 = Interpolate 1D Array(1:w549, 2:w538) -> (0:w547:dbl)
        n260 = Subtract(x=w507, y=w506) -> (x-y=w505:dbl)
        n261 = Subtract(x=w548, y=w547) -> (x-y=w546:dbl)
        n262 = Absolute Value(x=w505) -> (abs(x)=w500:dbl)
        n263 = Absolute Value(x=w546) -> ()  [unwired: 1 out]
        n264 = In Range and Coerce(upper limit=w543, x=w500, lower limit=w544) -> (In Range?=w540:bool)  [unwired: 1 out]
        n265 = Select(t="OK", s=w540, f="NG") -> (s? t:f=w539:string)
      }
      frame 18 {
        # "监测点3主信号滞后"
        n266 = Index Array(array=w581, index #1=7 ("索引"), index #2=10 ("索引"), index #3=1 ("索引"), index #4=4 ("索引")) -> (element #1=w599:cluster{"X":dbl[], "Y":dbl[]}, element #2=w598:cluster{"X":dbl[], "Y":dbl[]}, element #3=w595:cluster{"X":dbl[], "Y":dbl[]}, element #4=w594:cluster{"X":dbl[], "Y":dbl[]})
        n267 = Index Array(array=w581, index #1=1 ("索引"), index #2=7 ("索引"), index #3=4 ("索引"), index #4=10 ("索引")) -> (element #1=w576:cluster{"X":dbl[], "Y":dbl[]}, element #2=w575:cluster{"X":dbl[], "Y":dbl[]}, element #3=w574:cluster{"X":dbl[], "Y":dbl[]}, element #4=w573:cluster{"X":dbl[], "Y":dbl[]})
        n268 = global read "Global.vi" "复检参数"() -> (w616:T3)
        n269 = Unbundle(w598) -> ("X"=w593:dbl[], "Y"=w592:dbl[])
        n270 = Unbundle(w595) -> ("X"=w591:dbl[], "Y"=w590:dbl[])
        n271 = Unbundle(w594) -> ("X"=w589:dbl[], "Y"=w588:dbl[])
        n272 = Unbundle(w599) -> ("X"=w587:dbl[], "Y"=w586:dbl[])
        n273 = Unbundle(w576) -> ("X"=w572:dbl[], "Y"=w570:dbl[])
        n274 = Unbundle(w575) -> ("X"=w571:dbl[], "Y"=w569:dbl[])
        n275 = Unbundle(w574) -> ("X"=w564:dbl[], "Y"=w562:dbl[])
        n276 = Unbundle(w573) -> ("X"=w563:dbl[], "Y"=w561:dbl[])
        n277 = Unbundle By Name(w616) -> ("滞后监测点3"=w557:dbl)
        n278 = Build Array (concatenate)(w593, w591) -> (w585:dbl[])
        n279 = Build Array (concatenate)(w592, w590) -> (w584:dbl[])
        n280 = Build Array (concatenate)(w589, w587) -> (w583:dbl[])
        n281 = Build Array (concatenate)(w588, w586) -> (w582:dbl[])
        n282 = Build Array (concatenate)(w570, w569) -> (w568:dbl[])
        n283 = Build Array (concatenate)(w572, w571) -> (w567:dbl[])
        n284 = Build Array (concatenate)(w564, w563) -> (w560:dbl[])
        n285 = Build Array (concatenate)(w562, w561) -> (w559:dbl[])
        n286 = Reverse 1D Array(array=w559) -> (reversed array=w558:dbl[])
        n287 = Threshold 1D Array(2:w557, 3:w584) -> (0:w615:dbl)  [unwired: 1 in]
        n288 = Reverse 1D Array(array=w583) -> (reversed array=w602:dbl[])
        n289 = Reverse 1D Array(array=w582) -> (reversed array=w614:dbl[])
        n290 = Reverse 1D Array(array=w560) -> (reversed array=w556:dbl[])
        n291 = Threshold 1D Array(2:w557, 3:w568) -> (0:w566:dbl)  [unwired: 1 in]
        n292 = Interpolate 1D Array(1:w615, 2:w585) -> (0:w612:dbl)
        n293 = Threshold 1D Array(2:w557, 3:w614) -> (0:w613:dbl)  [unwired: 1 in]
        n294 = Interpolate 1D Array(1:w566, 2:w567) -> (0:w565:dbl)
        n295 = Threshold 1D Array(2:w557, 3:w558) -> (0:w555:dbl)  [unwired: 1 in]
        n296 = Interpolate 1D Array(1:w613, 2:w602) -> (0:w611:dbl)
        n297 = Interpolate 1D Array(1:w555, 2:w556) -> (0:w554:dbl)
        n298 = Subtract(x=w612, y=w611) -> ()  [unwired: 1 out]
        n299 = Subtract(x=w565, y=w554) -> (x-y=w553:dbl)
        n300 = Absolute Value(x=w553) -> (abs(x)=w607:dbl)
        n301 = In Range and Coerce(upper limit=w608, x=w607, lower limit=w609) -> (In Range?=w604:bool)  [unwired: 1 out]
        n302 = Select(t="OK", s=w604, f="NG") -> (s? t:f=w603:string)
      }
      frame 19 {
        # "监测点3副信号滞后"
        n303 = Index Array(array=w621, index #1=6 ("索引"), index #2=9 ("索引"), index #3=0 ("索引"), index #4=3 ("索引")) -> (element #1=w635:cluster{"X":dbl[], "Y":dbl[]}, element #2=w634:cluster{"X":dbl[], "Y":dbl[]}, element #3=w631:cluster{"X":dbl[], "Y":dbl[]}, element #4=w630:cluster{"X":dbl[], "Y":dbl[]})
        n304 = global read "Global.vi" "复检参数"() -> (w654:T3)
        n305 = Unbundle(w634) -> ("X"=w629:dbl[], "Y"=w628:dbl[])
        n306 = Unbundle(w631) -> ("X"=w627:dbl[], "Y"=w626:dbl[])
        n307 = Unbundle(w630) -> ("X"=w625:dbl[], "Y"=w624:dbl[])
        n308 = Unbundle(w635) -> ("X"=w623:dbl[], "Y"=w622:dbl[])
        n309 = Unbundle By Name(w654) -> ("滞后监测点3"=w651:dbl)
        n310 = Build Array (concatenate)(w629, w627) -> (w620:dbl[])
        n311 = Build Array (concatenate)(w628, w626) -> (w619:dbl[])
        n312 = Build Array (concatenate)(w625, w623) -> (w618:dbl[])
        n313 = Build Array (concatenate)(w624, w622) -> (w617:dbl[])
        n314 = Threshold 1D Array(2:w651, 3:w619) -> (0:w653:dbl)  [unwired: 1 in]
        n315 = Reverse 1D Array(array=w618) -> (reversed array=w638:dbl[])
        n316 = Reverse 1D Array(array=w617) -> (reversed array=w652:dbl[])
        n317 = Interpolate 1D Array(1:w653, 2:w620) -> (0:w649:dbl)
        n318 = Threshold 1D Array(2:w651, 3:w652) -> (0:w650:dbl)  [unwired: 1 in]
        n319 = Interpolate 1D Array(1:w650, 2:w638) -> (0:w648:dbl)
        n320 = Subtract(x=w649, y=w648) -> (x-y=w647:dbl)
        n321 = Absolute Value(x=w647) -> (abs(x)=w643:dbl)
        n322 = In Range and Coerce(upper limit=w644, x=w643, lower limit=w645) -> (In Range?=w640:bool)  [unwired: 1 out]
        n323 = Select(t="OK", s=w640, f="NG") -> (s? t:f=w639:string)
      }
    }
    n324 = Number To Fractional String(number=w27, precision (6)=w34) -> (F-format string=w33:string)  [unwired: 2 in]
    n325 = Number To Fractional String(number=w26, precision (6)=w34) -> (F-format string=w31:string)  [unwired: 2 in]
    n326 = Number To Fractional String(number=w36, precision (6)=w34) -> (F-format string=w32:string)  [unwired: 2 in]
    n327 = Build Array(w33, w32, w31, w28, w30) -> (w25:string[])
  }
  n328 = property class="Tbl"(reference="Result") -> (reference out=w10:refnum<vi>, error out=w15:errorcluster, "Row Headers[]"=w6:string[])  [unwired: 1 in]
  n329 = And Array Elements(Boolean array=w2) -> (logical AND=→"OK？":bool)
  n330 = Array Size(array=w2) -> (size(s)=w1:i32)
  n331 = Build Array (concatenate)(w6, "传感器特性" ("Label.Text"), w8) -> (w9:string[])
  n332 = global write "检测结果.vi" "传感器特性长度"(w1) -> ()
  n333 = property class="Tbl"(reference=w10, error in=w15, "Row Headers[]"=w9) -> (reference out=w11:refnum<vi>, error out=w14:errorcluster)
  n334 = property class="Tbl"(reference=w11, error in=w14) -> (reference out=w12:refnum<vi>, error out=w13:errorcluster, "Value"=w16:string[][])
  n335 = Build Array (concatenate)(w16, string[] ["", "", "", "", ""], w4) -> (w17:string[][])
  n336 = property class="Tbl"(reference=w12, error in=w13, "Value"=w17) -> ()  [unwired: 2 out]
